vi "Questao2VF_Ulisses_PEE.vi"() -> ()   [LabVIEW 2019]
uses:
  <vilib>/measure/matone.llb/Extract Single Tone Information 1 Chan.vi
  <vilib>/measure/NI_MAPro.lvlib
panel:
  out "Elevação":bool
  out "Afundamento":bool
  out "Interrupção":bool
  out "Regime":bool
  in  "Path":path
  out "Y max":dbl format="%0.2f"
  out "Waveform Graph 2":dbl[](graph)
  out "detected amplitude":dbl format="%.2p"
  out "dt":dbl
  out "size(s)":i32
  out "Sinal completo":waveform(dbl)(graph)
  # "Phase em graus"
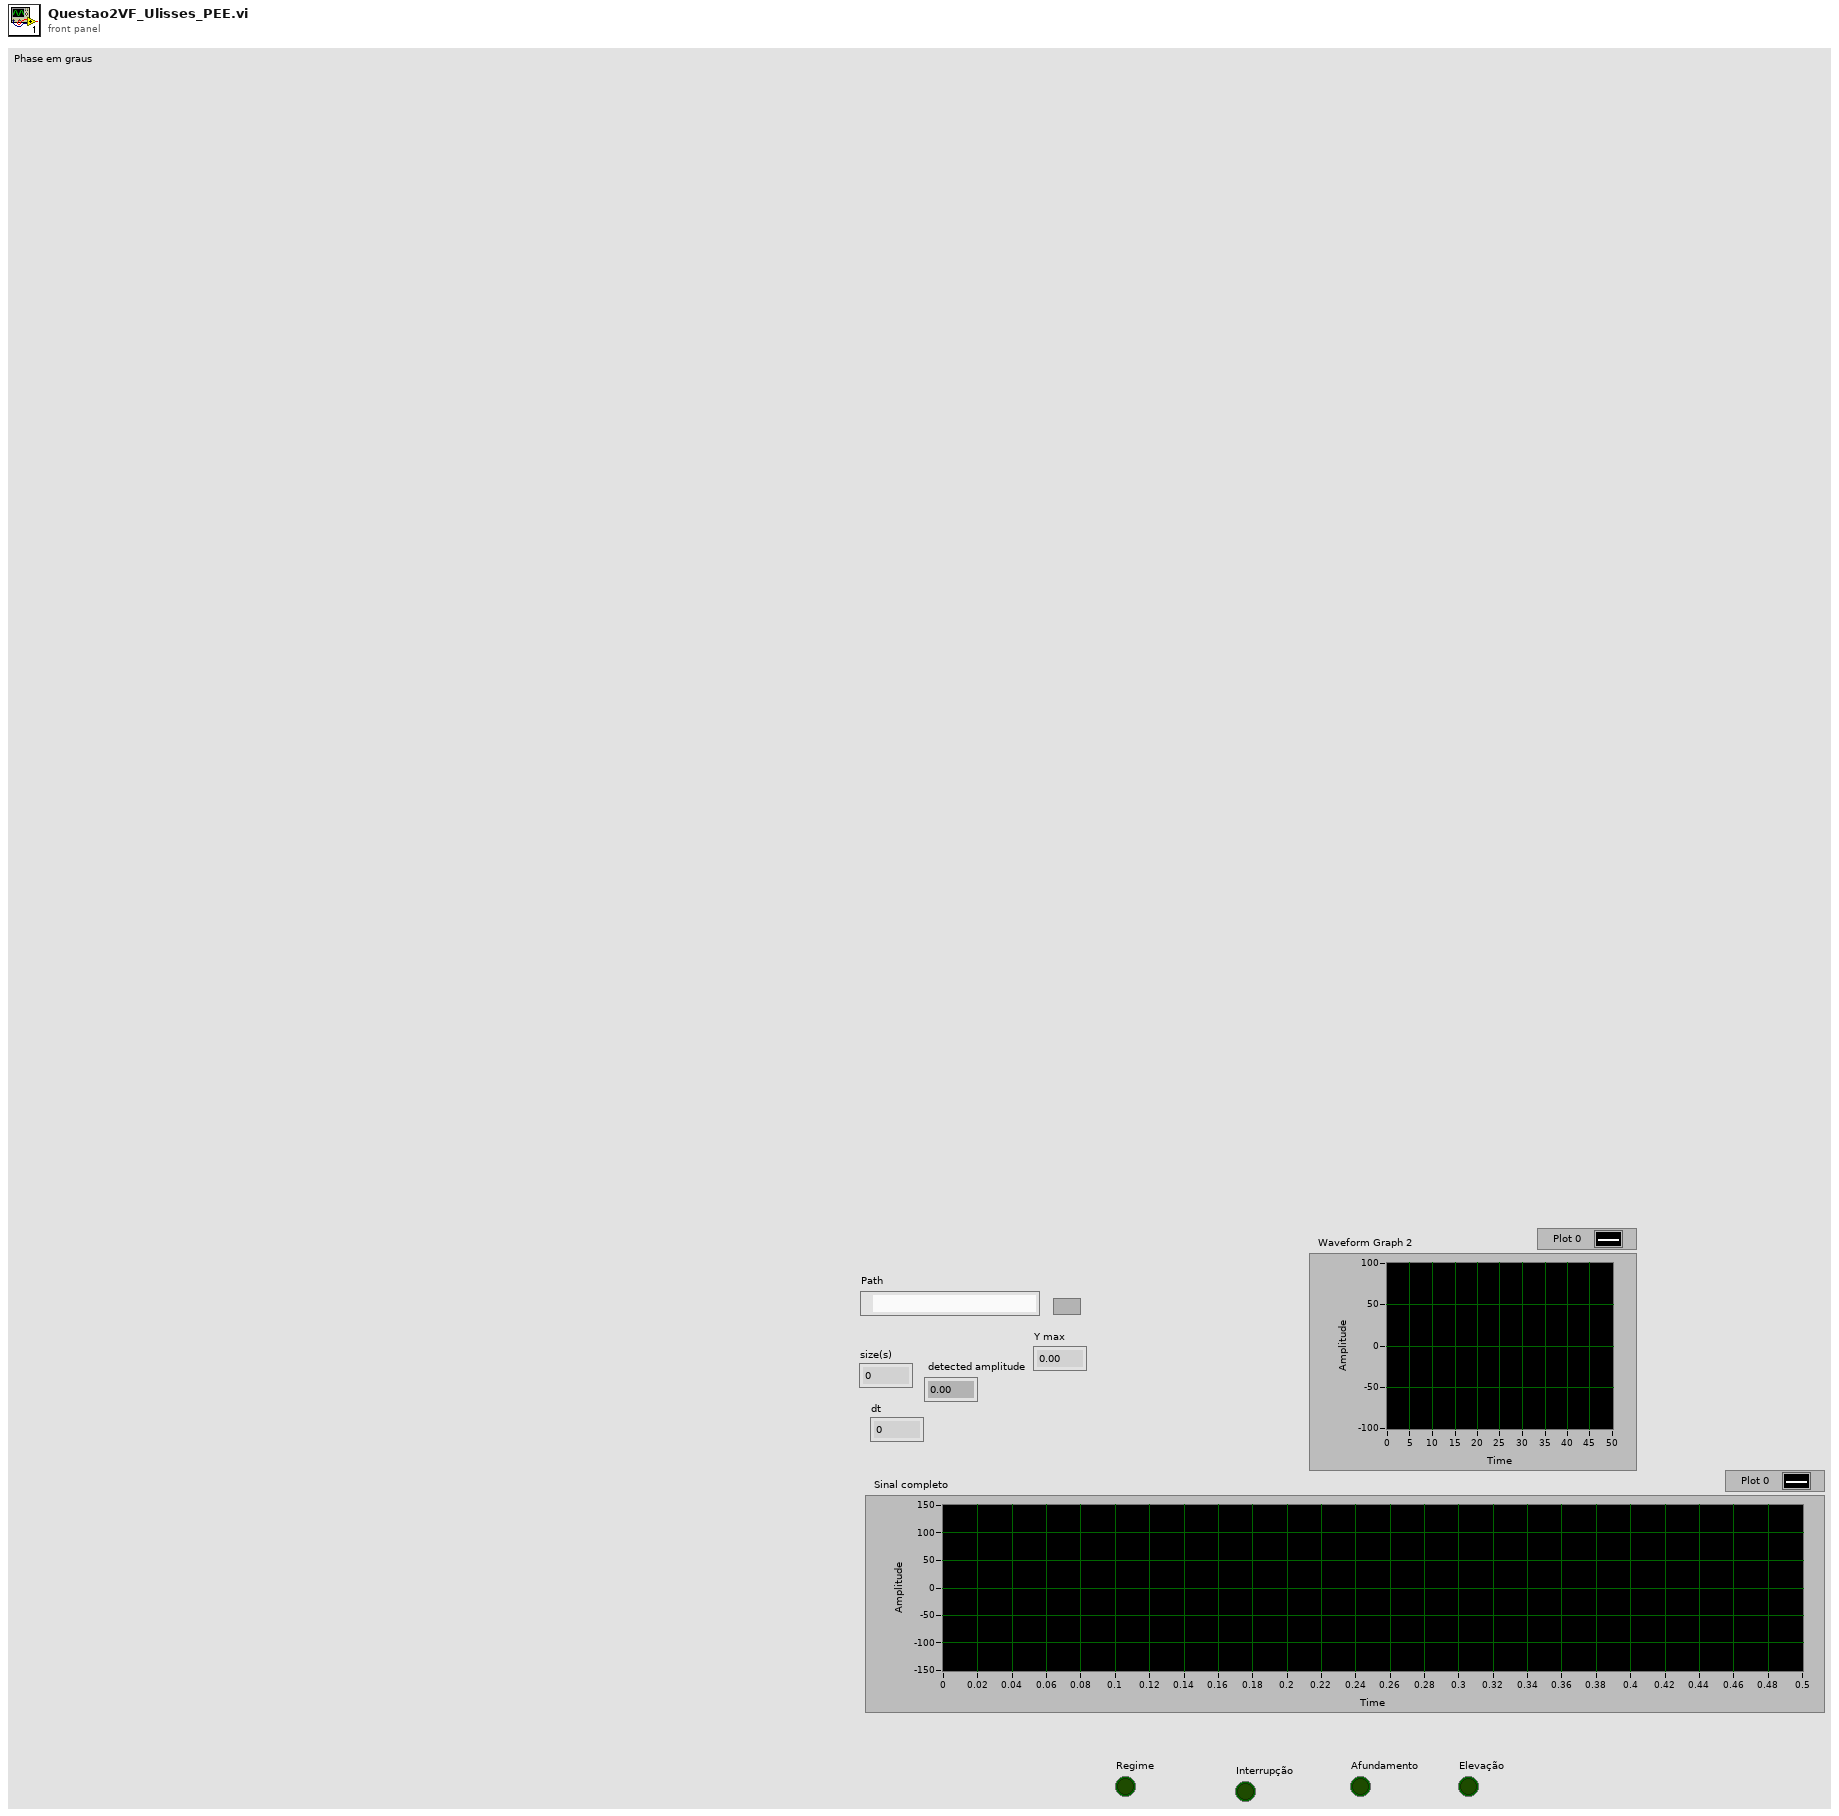
[diagram p1: front panel]
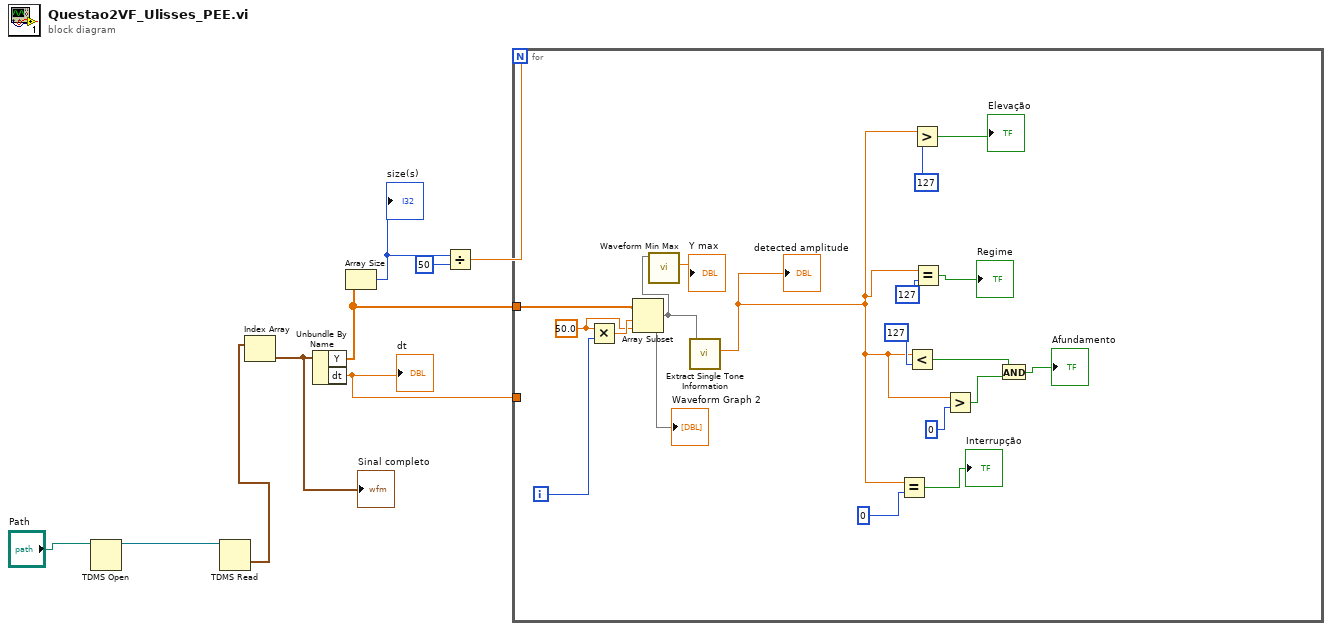
[diagram p0: block diagram]
diagram:
  n1 = TDMS Open(11:"Path") -> (3:w9:refnum<k34>)  [unwired: 6 in, 1 out]
  n2 = TDMS Read(0:w9) -> (10:w8:waveform(dbl)[])  [unwired: 7 in, 5 out]
  n3 = Index Array(array=w8) -> (element=w7:waveform(dbl))  [unwired: 1 in]
  "Sinal completo" <- w7
  n4 = Unbundle By Name(w7) -> ("Y"=w3:dbl[], "dt"=w4:dbl)
  "dt" <- w4
  n5 = Array Size(array=w3) -> (size(s)=w6:i32)
  "size(s)" <- w6
  n6 = Divide(x=w6, y=50) -> (x/y=w1:dbl)
  n7 = for {
    N: w1 -> [_]
    tunnel: w3 -> [w27]
    tunnel: w4 -> [_]
    i -> [w26]
    w24 = 50.0 ("x")
    n8 = Multiply(x=w24, y=w26) -> (x*y=w25:dbl)
    n9 = Array Subset(array=w27, index=w25, length=w24) -> (w22:dbl[])
    "Waveform Graph 2" <- w22
    n10 = call <vilib>:"Waveform Min Max.vi"("waveform in"=w22) -> ("Y max"=→"Y max":dbl)  [unwired: 5 in, 5 out]
    n11 = call-poly <vilib>:"Extract Single Tone Information.vi"("time signal in"=w22) -> ("detected amplitude"=w15:dbl)  [unwired: 5 in, 5 out]
    "detected amplitude" <- w15
    n12 = Equal?(x=w15, y=0) -> (x = y?=→"Interrupção":bool)
    n13 = Less?(x=w15, y=127) -> (x < y?=w18:bool)
    n14 = Greater?(x=w15, y=127) -> (0:→"Elevação":bool)
    n15 = Equal?(x=w15, y=127) -> (x = y?=→"Regime":bool)
    n16 = Greater?(x=w15, y=0) -> (0:w16:bool)
    n17 = And(x=w18, y=w16) -> (x .and. y?=→"Afundamento":bool)
  }
